vi "RT_Main_R1.vi"() -> ()   [LabVIEW 2018]
uses:
  <vilib>/Platform/TimedLoop/XDataNode/timing_clust.ctl
  <vilib>/Platform/TimedLoop/XDataNode/nitl_modes.ctl
  <vilib>/Platform/TimedLoop/XDataNode/wakeup.ctl
  <vilib>/FPGAPlugInAG/sbRIO-9606/niLvFpga_Open_sbRIO-9606.vi
  <vilib>/rvi/interface/common/dynamic/niFpgaDynamicAddResources.vi
  <vilib>/Utility/error.llb/Error Cluster From Error Code.vi
  <vilib>/rvi/errors/niLvFpgaAdjustHostInterfaceError.vi
  <vilib>/FPGAPlugInAG/Dynamic/niLvFpga_Close_Dynamic.vi
  <vilib>/rvi/interface/nirviOpenFPGA/nirviOpenFPGA.xnode
  FPGA/Bitfile/FPGA_Main_R3.lvbitx
  <vilib>/rvi/interface/nirviMethod/nirviMethod.xnode
  <vilib>/Platform/TimedLoop/XDataNode/XDataNode.xnode
  <vilib>/rvi/interface/nirviReadWriteControl/nirviReadWriteControl.xnode
  <vilib>/rvi/interface/nirviCloseFPGA/nirviCloseFPGA.xnode
  NiFpgaLv.dll
  <vilib>/rvi/interface/Simulation/niFpgaSimulationCallBeginRW.vi
  <vilib>/FPGAPlugInAG/Dynamic/niLvFpga_ReadFifo_Dynamic.vi
  <vilib>/rvi/errors/niLvFpgaMergeErrorWithErrorCode.vi
  <vilib>/Platform/TimedLoop/XDataNode/XDNodeRunTimeDep.lvlib
panel:
  out "Iteration Duration":i64
  out "Elements Remaining":u32
  in  "stop":bool
  out "Waveform Chart":T1(graph)
  out "Data Out":T1
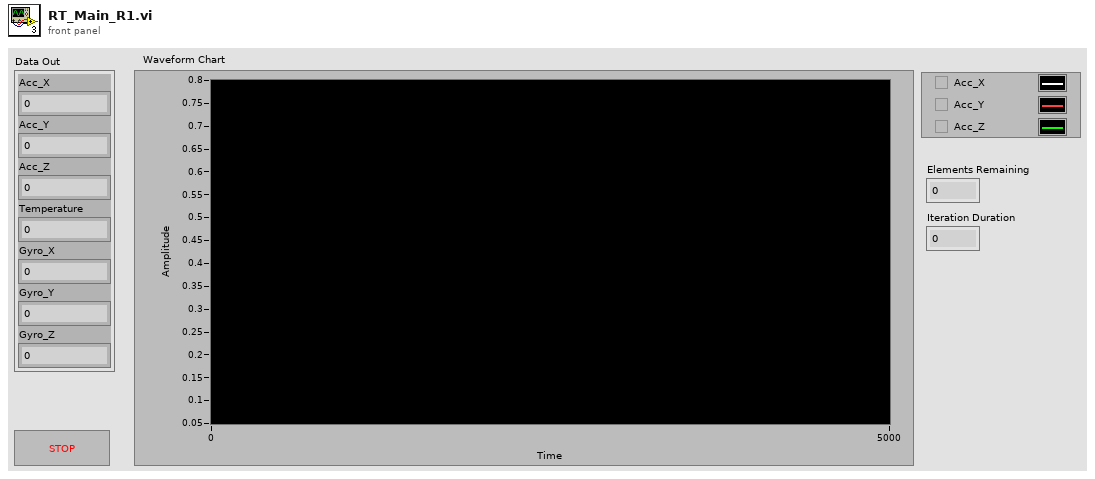
[diagram p1: front panel]
types:
  T1 = cluster{"Acc_X":dbl, "Acc_Y":dbl, "Acc_Z":dbl, "Temperature":dbl, "Gyro_X":dbl, "Gyro_Y":dbl, "Gyro_Z":dbl}
  T2 = typedef "XDNodeRunTimeDep.lvlib/timing_clust.ctl" = cluster{"Expected End [f-1]":u64, "Actual End [f-1]":u64, "Finished Late? [f-1]":bool, "Expected End [i-1]":u64, "Actual End [i-1]":u64, "Finished Late? [i-1]":bool, "Expected Start [i]":u64, "Actual Start [i]":u64, "Expected Start [f]":u64, "Actual Start [f]":u64, "Source Name":string, "Structure Name":string, "Period":i64, "Deadline":i64, "Offset":i64, "Start":i64, "Priority":i32, "Timeout":i32, "Mode":T3, "Wakeup Reason":T4, "Error":errorcluster, "Source Type":string, "Secondary Source Type":string, "Global End Time":u64, "Global Start Time":u64, "Frame Duration":u64, "Iteration Duration":u64, "Assigned CPU":i32, "I/O Scan Engine Mode":u32}
  T3 = typedef "XDNodeRunTimeDep.lvlib/nitl_modes.ctl" = enum32{"No Change", "Process missed periods, maintain original phase", "Discard missed periods, maintain original phase", "Process missed periods, ignore original phase", "Discard missed periods, ignore original phase"}
  T4 = typedef "XDNodeRunTimeDep.lvlib/wakeup.ctl" = enum32{"Normal", "Aborted", "Asynchronous wakeup", "Timing source error", "Timed loop error", "Timeout"}
  T5 = enum16{"Idle", "Set Idle", "Config", "Read", "Write", "Arm", "Auto Run", "Auto Config", "Auto Write", "Auto Arm", "Auto Read", "Auto Check"}
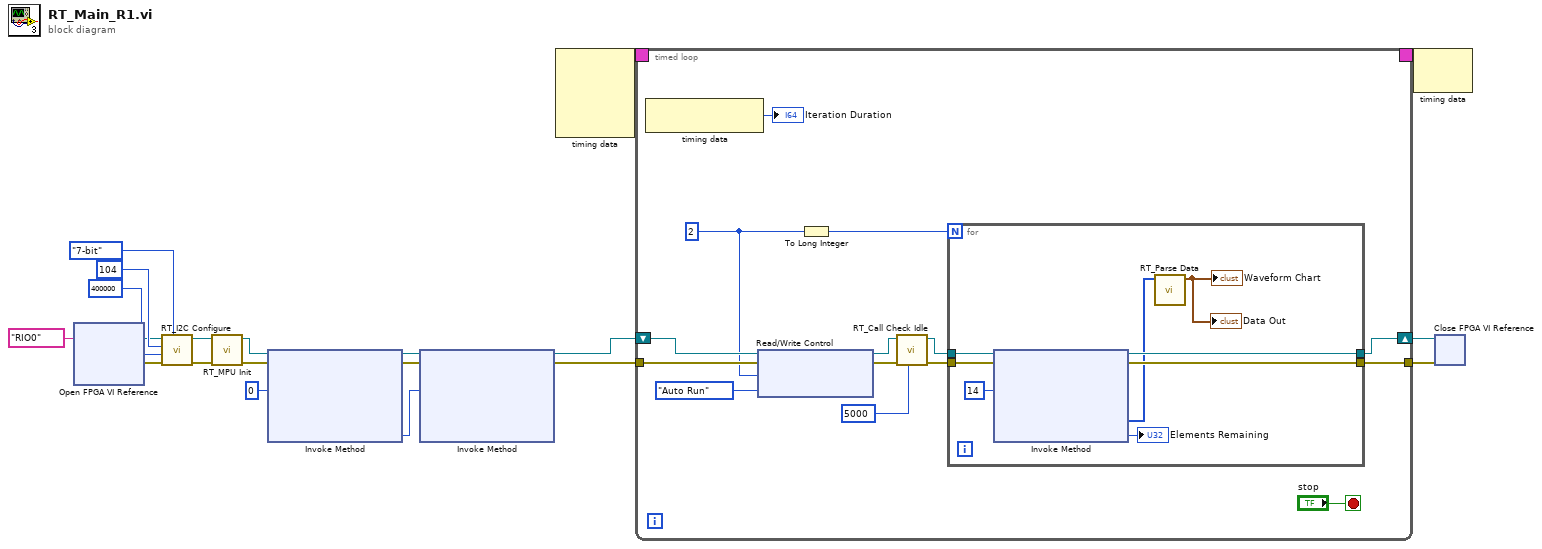
[diagram p0: block diagram]
diagram:
  n1 = xnode "Open FPGA VI Reference"("resource name"=tag "RIO0") -> ("FPGA VI Reference Out"=w11:refnum<k20>, "error out"=w19:errorcluster)  [unwired: 1 in]
  n2 = call "RT_I2C Configure.vi"("Address Type (7-bit)"=enum16{"7-bit", "10-bit"}."7-bit", "error in"=w19, "Clock Rate"=u32 400000, "IICSlaveAddress"=u16 104, "FPGA VI Reference In"=w11) -> ("error out"=w15:errorcluster, "FPGA VI Reference Out"=w14:refnum<k20>)  [unwired: 5 in]
  n3 = call "RT_MPU Init.vi"("error in"=w15, "FPGA VI Reference In"=w14) -> ("error out"=w10:errorcluster, "FPGA VI Reference Out"=w9:refnum<k20>)  [unwired: 8 in]
  n4 = xnode "Invoke Method"("FPGA VI Reference In"=w9, "error in"=w10, "Number of Elements"=u32 0) -> ("FPGA VI Reference Out"=w6:refnum<k20>, "error out"=w7:errorcluster, "Elements Remaining"=w5:u32)  [unwired: 1 in, 1 out]
  n5 = xnode "Invoke Method"("FPGA VI Reference In"=w6, "error in"=w7, "Number of Elements"=w5) -> ("FPGA VI Reference Out"=w3:refnum<k20>, "error out"=w4:errorcluster)  [unwired: 1 in, 2 out]
  n6 = node-c288() -> (w2:T2)  [unwired: 4 in]
  n7 = timed-loop {
    shift-right: [w31] -> w12
    shift-left: w3 -> [w34]
    tunnel: w4 -> [w33]
    tunnel: [w32] -> w13
    timing: w2 -> [_]
    timing-out: [_] -> w1
    stop <- "stop" stop-if-true
    w24 = u32 2 ("Auto Read Count")
    n8 = node-c288() -> (→"Iteration Duration":i64)  [unwired: 1 in]
    n9 = xnode "Read/Write Control"("FPGA VI Reference In"=w34, "error in"=w33, "Auto Read Count"=w24, "I2C Loop State"=T5."Auto Run") -> ("FPGA VI Reference Out"=w26:refnum<k20>, "error out"=w27:errorcluster)
    n10 = To Long Integer(number=w24) -> (32bit integer=w23:i32)
    n11 = call "RT_Call Check Idle.vi"("Timeout?"=5000, "error in"=w27, "FPGA VI Reference In"=w26) -> ("error out"=w25:errorcluster, "FPGA VI Reference Out"=w22:refnum<k20>)  [unwired: 7 in]
    n12 = for {
      N: w23 -> [_]
      tunnel: [w43] -> w31
      tunnel: w25 -> [w42]
      tunnel: [w44] -> w32
      tunnel: w22 -> [w41]
      n13 = xnode "Invoke Method"("FPGA VI Reference In"=w41, "error in"=w42, "Number of Elements"=u32 14) -> ("FPGA VI Reference Out"=w43:refnum<k20>, "error out"=w44:errorcluster, "Data"=w38:u8[], "Elements Remaining"=→"Elements Remaining":u32)  [unwired: 1 in]
      n14 = call "RT_Parse Data.vi"("Data In"=w38) -> ("Data Out"=→"Data Out" →"Waveform Chart":T1)  [unwired: 10 in]
    }
  }
  n15 = node-c288(w1) -> ()  [unwired: 1 out]
  n16 = xnode "Close FPGA VI Reference"("FPGA VI Reference In"=w12, "error in"=w13) -> ()  [unwired: 1 out]
